vi "NewPort_PM_USB_Cmd.vi"(8 "error in":errorcluster, 9 "PM:CMD_QUERY In":string, 10 "USB Address":i32, 11 "reference":refnum<k24>) -> (0 "Error Out":errorcluster, 2 "Query-Double\nfrom Read Buffer\nFirst Info":dbl, 3 "Query-String\nfrom Read Buffer\nComplete Info":string)   [LabVIEW 2017]
uses:
  C:/Program Files (x86)/Newport/Newport USB Driver/Bin/UsbDllWrap.dll
  Program Files (x86)/Newport/Newport USB Driver/Bin/UsbDllWrap.dll
panel:
  out "Read":i32
  # "Model 1931-C|1936-C = Single Channel\nModel 2936-R = Dual Channel"
  # "This enables wavelength setting on and power reading from the power meter"
  # "Input"
  # "Output"
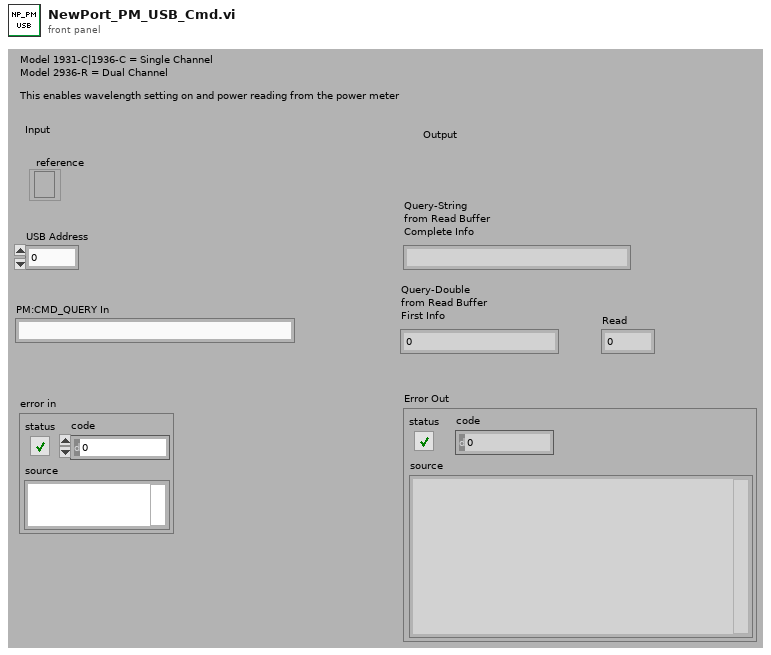
[diagram p1: front panel]
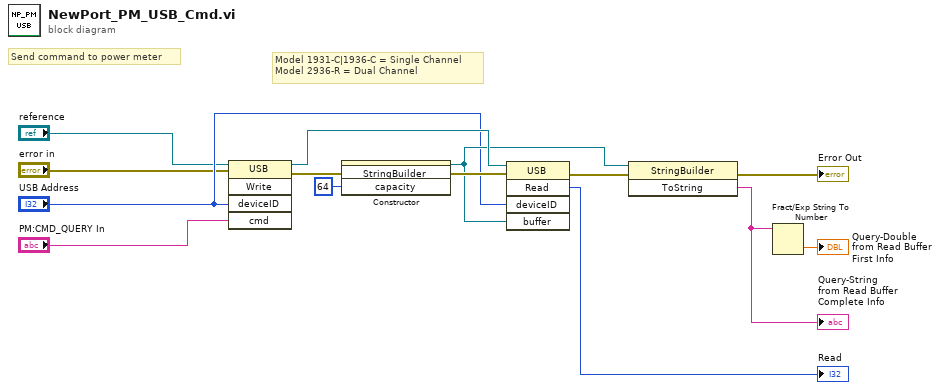
[diagram p0: block diagram]
diagram:
  # "Send command to power meter"
  # "Model 1931-C|1936-C = Single Channel\nModel 2936-R = Dual Channel"
  n1 = invoke class="USB" method="Write"(reference="reference", error in="error in", "deviceID"="USB Address", "cmd"="PM:CMD_QUERY In") -> (reference out=w11:refnum<k24>, error out=w14:errorcluster)  [unwired: 1 in, 3 out]
  n2 = constructor class="StringBuilder"(error in=w14, "capacity"=64) -> (reference out=w10:refnum<k24>, error out=w12:errorcluster)  [unwired: 2 in, 2 out]
  n3 = invoke class="USB" method="Read"(reference=w11, error in=w12, "deviceID"="USB Address", "buffer"=w10) -> (error out=w9:errorcluster, "Read"=→"Read":i32)  [unwired: 1 in, 3 out]
  n4 = invoke class="StringBuilder" method="ToString"(reference=w10, error in=w9) -> (error out=→"Error Out":errorcluster, "ToString"=w3:string)  [unwired: 1 in, 1 out]
  "Query-String\nfrom Read Buffer\nComplete Info" <- w3
  n5 = Fract/Exp String To Number(string=w3) -> (number=→"Query-Double\nfrom Read Buffer\nFirst Info":dbl)  [unwired: 3 in, 1 out]
